vi "Handle Command.vi"(8 "error in":errorcluster, 10 "Change Speaker State in":refnum<class "Change Speaker State.lvclass">, 11 "Object In":refnum<class>) -> (0 "error out":errorcluster, 1 "Command Successful?":bool, 2 "Change Speaker State out":refnum<class "Change Speaker State.lvclass">, 3 "Object Out":refnum<class>)   [LabVIEW 2018, in "ePAS Library.lvlib" / "Change Speaker State.lvclass"]
doc: "Change the current speaker position, log that position if the command is good (record the error if it is not) and update the data object."
uses:
  Change Speaker State.lvclass
  FPGA/Session/Exscalabar FPGA.lvclass
  Instrument/ePAS.lvclass
  C:/Users/Labview/Documents/exscalabar_server/reusable/Instrument/Instrument.lvclass
  C:/Users/Labview/Documents/exscalabar_server/reusable/PAS/Main/PAS.lvclass
  reusable/PAS/Data/Main/PAS Data.lvclass
  C:/Users/Labview/Documents/exscalabar_server/reusable/Data/Data.lvclass
  Instrument/ePAS.lvclass/ePAS.ctl
  reusable/Instrument/Instrument.lvclass/Instrument.ctl
  Change Speaker State.lvclass/Change Speaker State.ctl
  Change PAS Laser Frequency/Change Laser Frequency.lvclass
  C:/Users/Labview/Documents/exscalabar_server/reusable/Command/Command.lvclass
  Change PAS Laser Frequency/Change Laser Frequency.lvclass/Change Laser Frequency.ctl
  FPGA/Session/Exscalabar FPGA.lvclass/Exscalabar FPGA.ctl
  Change PAS Laser Frequency/Write f0.vi
  <vilib>/DAQmx/write.llb/DAQmx Write (Digital Bool 1Line 1Point).vi
  Instrument/Accessors/Read FPGA Session.vi
  reusable/Instrument/Read Data.vi
  reusable/Instrument/Read Log Session.vi
  reusable/Instrument/Read CMD.vi
  FPGA/Session/Read Ex FPGA Ref.vi
  reusable/Instrument/Write Data.vi
  reusable/PAS/Main/Read Switch Ref.vi
  <vilib>/Utility/error.llb/Error Cluster From Error Code.vi
  <vilib>/rvi/errors/niLvFpgaAdjustHostInterfaceError.vi
  reusable/PAS/Data/Main/Write drive.vi
  reusable/PAS/Data/Main/Read CellData.vi
  reusable/PAS/Main/Set Speaker Switch.vi
  reusable/PAS/Main/Write Speaker Reference.vi
  <vilib>/DAQmx/miscellaneous.llb/DAQmx Fill In Error Info.vi
  <userlib>/_Session Fwk/Session - Root.lvclass
  reusable/Data/Data.lvclass
  reusable/Switch/Switch.lvclass
  reusable/Command/Command.lvclass
  FPGA/R FPGA Ref.ctl
  <vilib>/rvi/interface/nirviReadWriteControl/nirviReadWriteControl.xnode
  FPGA Bitfiles/FPGAServer.lvbitx
  reusable/PAS/Data/Cell/PAS Cell Data.lvclass
  reusable/Session APIs/Session Log/System Log.lvclass
  ePAS Library.lvlib
  NiFpgaLv.dll
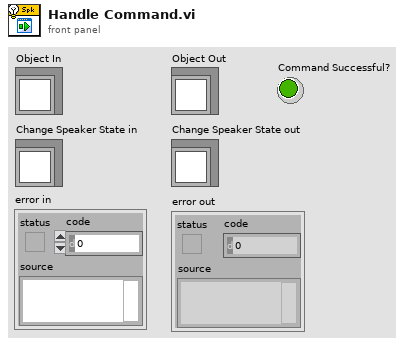
[diagram p1: front panel]
types:
  T1 = typedef "Session - Root.lvclass/Session Handle.ctl" = refnum<data-value>
  T2 = typedef "ePAS Library.lvlib/R FPGA Ref.ctl" = refnum<k20>
  T3 = cluster{"State":bool, "State":bool, "State":bool, "State":bool, "State":bool}
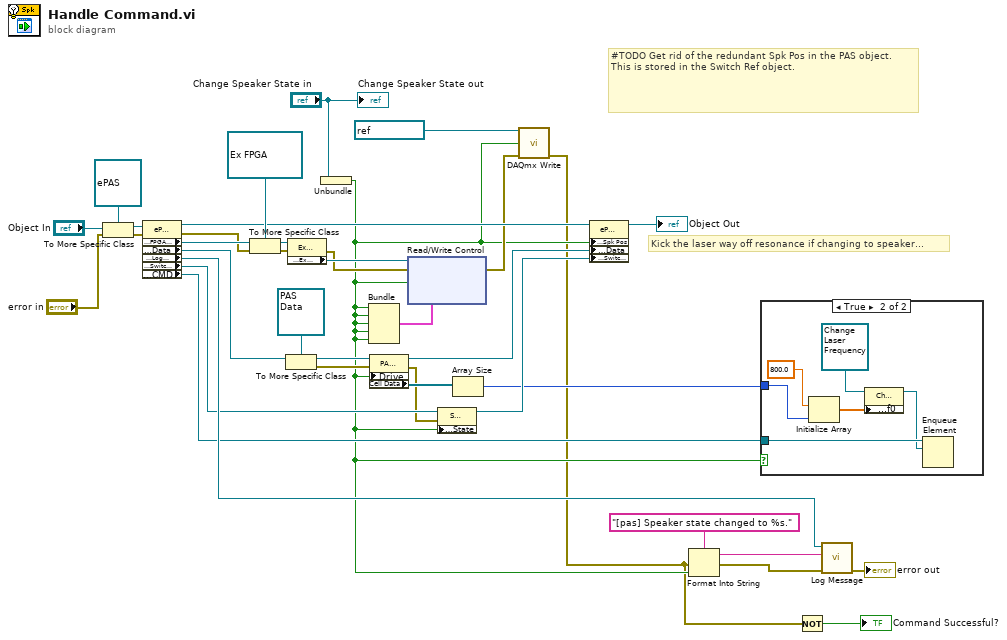
[diagram p0: block diagram]
diagram:
  # "Kick the laser way off resonance if changing to speaker..."
  # "#TODO Get rid of the redundant Spk Pos in the PAS object.  This is stored in the Switch Ref object."
  n1 = To More Specific Class(target class=refnum<class "ePAS.lvclass"> refnum ("ePAS.lvclass"), reference="Object In", error in="error in") -> (specific class reference=w33:refnum<class "ePAS.lvclass">, error out=w32:errorcluster)
  n2 = property class="ePAS"(reference=w33, error in=w32) -> (reference out=w19:refnum<class "ePAS.lvclass">, error out=w21:errorcluster, "Accessors:FPGA Session"=w30:T1, "Accessors:Data"=w29:refnum<class "Data.lvclass">, "Accessors:Log Session"=w25:T1, "Data Access:Switch Ref"=w18:refnum<class "Switch.lvclass">, "Accessors:CMD"=w8:refnum<queue>)
  n3 = To More Specific Class(target class=refnum<data-value> refnum ("Session Handle"), reference=w30, error in=w21) -> (specific class reference=w36:refnum<data-value>, error out=w35:errorcluster)
  n4 = To More Specific Class(target class=refnum<class "PAS Data.lvclass"> refnum ("PAS Data"), reference=w29) -> (specific class reference=w26:refnum<class "PAS Data.lvclass">, error out=w20:errorcluster)  [unwired: 1 in]
  n5 = property class="Ex FPGA"(reference=w36, error in=w35) -> (error out=w22:errorcluster, "Accessors:Ex FPGA Ref"=w27:T2)  [unwired: 1 out]
  n6 = Unbundle("Change Speaker State in") -> (w4:bool)
  n7 = Bundle("State"=w4, "State"=w4, "State"=w4, "State"=w4, "State"=w4) -> (w10:T3)  [unwired: 1 in]
  n8 = property class="PAS Data"(reference=w26, error in=w20, "Drive"=w4) -> (reference out=w5:refnum<class "PAS Data.lvclass">, error out=w3:errorcluster, "Cell Data"=w7:refnum<class "PAS Cell Data.lvclass">[])
  n9 = xnode "Read/Write Control"("FPGA VI Reference In"=w27, "error in"=w22, "Spk Enable"=w4, "iSpk Enable"=w10) -> ("error out"=w12:errorcluster)  [unwired: 1 out]
  n10 = property class="Switch"(reference=w18, error in=w3, "Data Access:State"=w4) -> (reference out=w17:refnum<class "Switch.lvclass">)  [unwired: 1 out]
  n11 = Array Size(array=w7) -> (size(s)=w6:i32)
  n12 = call-poly <vilib>:"DAQmx Write.vi"("task/channels in"=refnum<k21> "Spk LED", "data"=w4, "error in"=w12) -> ("error out"=w2:errorcluster)  [unwired: 10 in, 2 out]
  n13 = property class="ePAS"(reference=w19, "Data Access:Spk Pos"=w4, "Accessors:Data"=w5, "Data Access:Switch Ref"=w17) -> (reference out=→"Object Out":refnum<class "ePAS.lvclass">)  [unwired: 1 in, 1 out]
  n14 = Format Into String(format string="[pas] Speaker state changed to %s.", error in=w2, w4) -> (resulting string=w23:string, error out=w9:errorcluster)  [unwired: 1 in]
  n15 = case shown="True" w4 {
    tunnel: w8 -> [_ w42]
    tunnel: w6 -> [_ w41]
    frame False {
    }
    frame True {
      n16 = Initialize Array(800.0 ("element"), w41) -> (w40:dbl[])
      n17 = property class="Change Laser Frequency.lvclass"(reference=refnum<class "Change Laser Frequency.lvclass"> refnum ("ePAS Library.lvlib:Change Laser Frequency.lvclass"), "Accessors:f0"=w40) -> (reference out=w39:refnum<class "Change Laser Frequency.lvclass">)  [unwired: 1 in, 1 out]
      n18 = Enqueue Element(queue=w42, element=w39) -> ()  [unwired: 2 in, 3 out]
    }
  }
  n19 = Not(x=w2) -> (.not. x?=→"Command Successful?":bool)
  n20 = call "Log Message.vi"("error in"=w9, "MSG In"=w23, "session in"=w25) -> ("error out"=→"error out":errorcluster)  [unwired: 7 in, 1 out]
  "Change Speaker State out" <- "Change Speaker State in"
